vi "Set FP Size.vi"(8 "Error In":errorcluster, 9 "Position":cluster{"X":i16, "Y":i16}, 10 "Size":cluster{"Width":i16, "Height":i16}, 11 "VI Ref":refnum<vi>) -> (0 "Error Out":errorcluster)   [LabVIEW 2020, in "LMH-Toolbox.lvlib"]
doc: "Set the specified VIs front panel size and on screen position."
uses:
  LMH-Toolbox.lvlib
  <vilib>/Utility/miscctls.llb/LVRectTypeDef.ctl
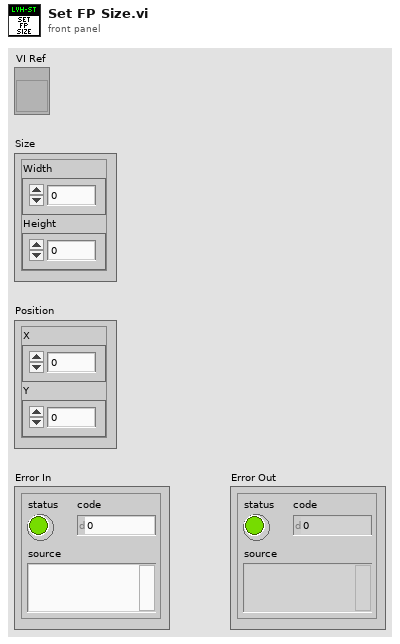
[diagram p1: front panel]
types:
  T1 = typedef "LVRectTypeDef.ctl" = cluster{"Left":i16, "Top":i16, "Right":i16, "Bottom":i16}
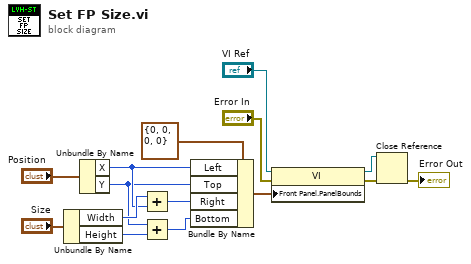
[diagram p0: block diagram]
diagram:
  n1 = Unbundle By Name("Size") -> ("Width"=w13:i16, "Height"=w10:i16)
  n2 = Unbundle By Name("Position") -> ("X"=w6:i16, "Y"=w5:i16)
  n3 = Add(x=w13, y=w6) -> (x+y=w12:i16)
  n4 = Add(x=w5, y=w10) -> (x+y=w11:i16)
  n5 = Bundle By Name(cluster=T1 {"Left"=0, "Top"=0, "Right"=0, "Bottom"=0} ("Front Panel Window:Panel Bounds"), "Left"=w6, "Top"=w5, "Right"=w12, "Bottom"=w11) -> (w1:T1)
  n6 = property class="VI"(reference="VI Ref", error in="Error In", "Front Panel.PanelBounds"=w1) -> (reference out=w9:refnum<vi>, error out=w8:errorcluster)
  n7 = Close Reference(reference=w9, error in (no error)=w8) -> (error out=→"Error Out":errorcluster)
